vi "Ophir_Measure.vi"(0 "INSTR_PARAM 2":refnum<vi>, 1 "error in (no error)":errorcluster) -> (2 "Overrange":bool, 3 "Power,uW":dbl, 4 "error out":errorcluster)   [LabVIEW 2012]
uses:
  Controls/Instr_Param.ctl
  TypeDefs/SMUParam.ctl
  Controls/USB4000_Data.ctl
  <vilib>/Analysis/NI_AALBase.lvlib
panel:
  out "Units":string
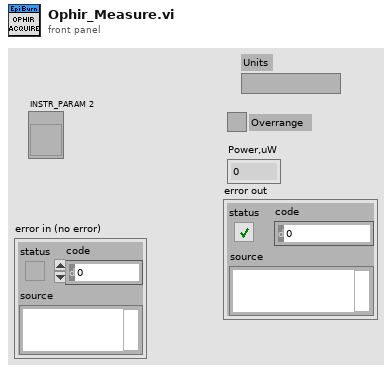
[diagram p1: front panel]
types:
  T1 = typedef "Instr_Param.ctl" = cluster{"Keithley_Param":T2, "USB4000_Param":cluster{"Integration Time":i32, "Wl min,nm":dbl, "Wl max,nm":dbl, "USB4000":T3}, "Ophir_Param":cluster{"VISA resource name":refnum<visa-resource-name>, "Calibration Wl":dbl}}
  T2 = typedef "SMUParam.ctl" = cluster{"Start Current,mA":dbl, "Stop Current,mA":dbl, "Voltage Compliance,V":dbl, "GPIB":string, "VISA resource name":refnum<visa-resource-name>}
  T3 = typedef "USB4000_Data.ctl" = cluster{"Wrapper Out":u32, "Number of Spectrometers":i32, "Wavelength":dbl[], "EL Spectrum":dbl[], "Int Time (usec)":i32, bool, "Background":dbl[]}
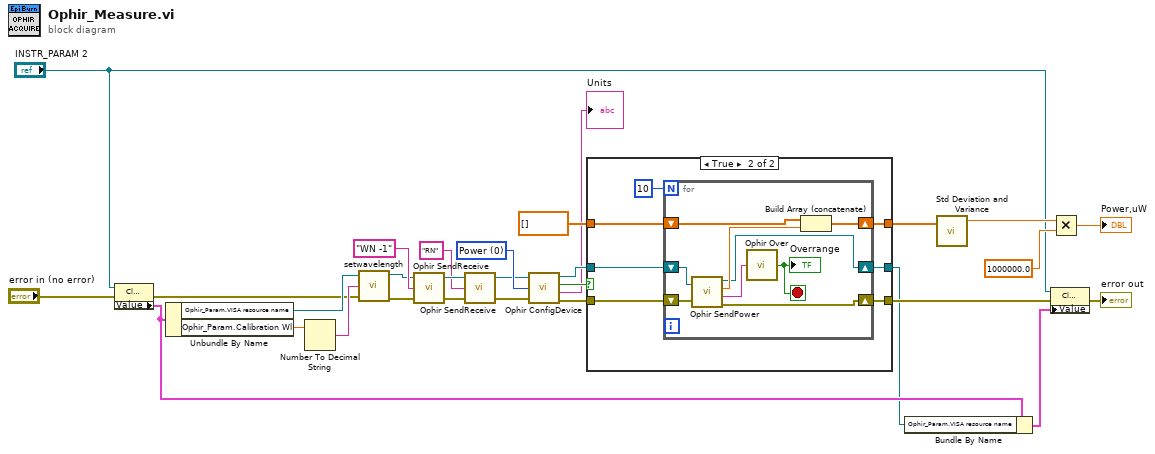
[diagram p0: block diagram]
diagram:
  w23 = u16 0 items=["Power", "Energy", "Frequency"] ("Measure Choice (0:Power)")
  n1 = property class="Clust (strict)"(reference="INSTR_PARAM 2", error in="error in (no error)") -> (error out=w9:errorcluster, "Value"=w4:T1)  [unwired: 1 out]
  n2 = Unbundle By Name(w4) -> ("Ophir_Param.VISA resource name"=w10:refnum<visa-resource-name>, "Ophir_Param.Calibration Wl"=w11:dbl)
  n3 = Number To Decimal String(number=w11) -> (decimal integer string=w12:string)  [unwired: 1 in]
  n4 = call "setwavelength.vi"("Dup Visa Session"=w10, "Set Wavelength"=w12, "error in (no error)"=w9) -> ("dup Visa Session"=w28:refnum<visa-resource-name>, "error out"=w27:errorcluster)  [unwired: 3 in]
  n5 = call "Ophir SendReceive.vi"("error in (no error)"=w27, "Command"="WN -1", "Visa Session"=w28) -> ("error out"=w24:errorcluster, "dup Visa Session"=w26:refnum<visa-resource-name>)  [unwired: 1 out]
  n6 = call "Ophir SendReceive.vi"("error in (no error)"=w24, "Command"="RN", "Visa Session"=w26) -> ("error out"=w21:errorcluster, "dup Visa Session"=w22:refnum<visa-resource-name>)  [unwired: 1 out]
  n7 = call "Ophir ConfigDevice.vi"("Visa Session"=w22, "Measure Choice (0:Power)"=w23, "error in (no error)"=w21) -> ("dup Visa Session"=w18:refnum<visa-resource-name>, "OK ?"=w20:bool, "Units"=→"Units":string, "error out"=w19:errorcluster)
  n8 = case shown="True" w20 {
    tunnel: w19 -> [w31 w37]
    tunnel: w18 -> [w32 w38]
    tunnel: dbl[] [] -> [w30 w39]
    tunnel: [w32 w36] -> w3
    tunnel: [w31 w35] -> w5
    tunnel: [w30 w34] -> w16
    frame False {
    }
    frame True {
      n9 = for {
        N: 10 -> [_]
        shift-right: [w42] -> w34
        shift-left: w39 -> [w48]
        shift-right: [w43] -> w36
        shift-left: w38 -> [w46]
        shift-right: [w44] -> w35
        shift-left: w37 -> [w45]
        stop <- w40 stop-if-true
        n10 = call "Ophir SendPower.vi"("Visa Session"=w46, "error in (no error)"=w45) -> ("dup Visa Session"=w43:refnum<visa-resource-name>, "Value Number"=w47:dbl, "Value String"=w41:string, "error out"=w44:errorcluster)
        n11 = call "Ophir Over.vi"("Value String"=w41) -> ("Overrange"=w40:bool)
        "Overrange" <- w40
        n12 = Build Array (concatenate)(w48, w47) -> (w42:dbl[])
      }
    }
  }
  n13 = Bundle By Name(cluster=w4, "Ophir_Param.VISA resource name"=w3) -> (w2:T1)
  n14 = call <vilib>:"Std Deviation and Variance.vi"("X"=w16) -> ("mean"=w14:dbl)  [unwired: 1 in, 2 out]
  n15 = Multiply(x=w14, y=1000000.0) -> (x*y=→"Power,uW":dbl)
  n16 = property class="Clust (strict)"(reference="INSTR_PARAM 2", error in=w5, "Value"=w2) -> (error out=→"error out":errorcluster)  [unwired: 1 out]
